vi "Packet Count from nRF52 String.vi"(8 "error in (no error)":errorcluster, 10 "Packet Count Info from nRF52":string="…Ü") -> (0 "error out":errorcluster, 2 "Returned Packet Count":u16)   [LabVIEW 2025]
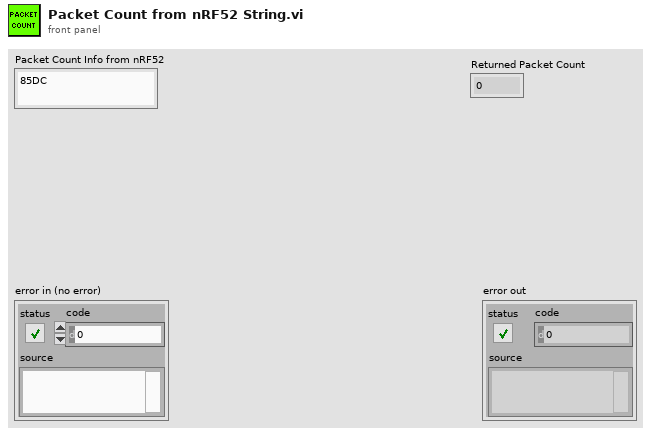
[diagram p1: front panel]
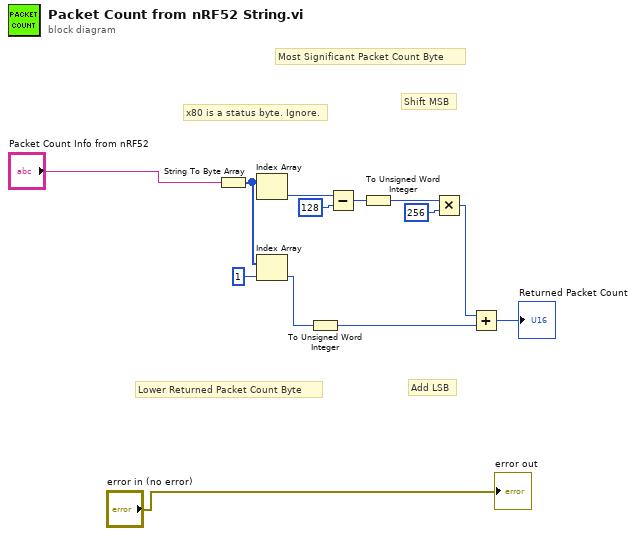
[diagram p0: block diagram]
diagram:
  # "Lower Returned Packet Count Byte"
  # "Add LSB"
  # "Shift MSB"
  # "Most Significant Packet Count Byte"
  # "x80 is a status byte. Ignore."
  n1 = String To Byte Array(string="Packet Count Info from nRF52") -> (unsigned byte array=w11:u8[])
  n2 = Index Array(array=w11) -> (element=w10:u8)  [unwired: 1 in]
  n3 = Index Array(array=w11, index=1) -> (element=w4:u8)
  n4 = To Unsigned Word Integer(number=w4) -> (unsigned 16bit integer=w3:u16)
  n5 = Subtract(x=w10, y=u8 128) -> (x-y=w8:u8)
  n6 = To Unsigned Word Integer(number=w8) -> (unsigned 16bit integer=w7:u16)
  n7 = Multiply(x=w7, y=u16 256) -> (x*y=w5:u16)
  n8 = Add(x=w5, y=w3) -> (x+y=→"Returned Packet Count":u16)
  "error out" <- "error in (no error)"
